vi "Create.vi"() -> (3 "EStop Identity out":refnum<class "EStop Identity.lvclass">)   [LabVIEW 2020, in "VolatusControl.lvlib" / "EStop Identity.lvclass"]
uses:
  EStop Identity.lvclass
  EStop Identity.lvclass/EStop Identity.ctl
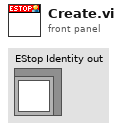
[diagram p1: front panel]
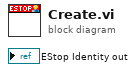
[diagram p0: block diagram]
diagram:
